vi "主动发送数据生成Condition(子VI).vi"(7 "结束时间":timestamp, 8 "数据发送协议":enum16{"2005-212协议", "2017-212协议"}(ring)=enum."2017-212协议", 9 "database":string, 10 "Label.Text":string, 11 "数值":i32) -> (0 "date/time string":string, 1 "database溢出":bool, 2 "columns":string[](array[string])=["时间", "测量模式", "数据类型", "检测值", "单位", "数据标识"], 3 "CONDITION":string)   [LabVIEW 2016, in "数据传输系统-02.lvlib"]
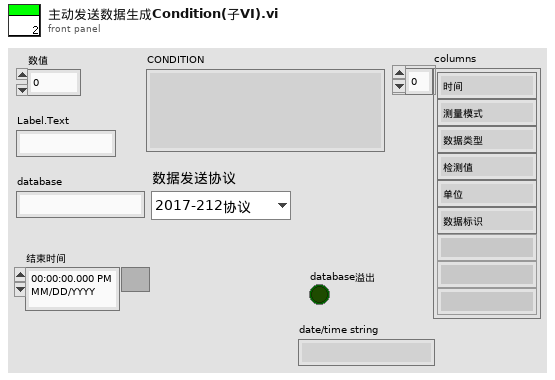
[diagram p1: front panel]
types:
  T1 = cluster{"time1":string, "time2":string, "time3":string, "time4":string, "time5":string, "time6":string, "time7":string, "time8":string, "time9":string, "time10":string, "time11":string, "time12":string, "time13":string, "time14":string, "time15":string, "time16":string, "time17":string, "time18":string, "time19":string, "time20":string, "time21":string, "time22":string, "time23":string, "time24":string, "time25":string, "time26":string, "time27":string, "time28":string, "time29":string, "time30":string, "time31":string, "time32":string, "time33":string, "time34":string, "time35":string, "time36":string, "time37":string, "time38":string, "time39":string, "time40":string, "time41":string, "time42":string, "time43":string, "time44":string, "time45":string, "time46":string, "time47":string, "time48":string, "time49":string, "time50":string, "time51":string, "time52":string, "time53":string, "time54":string, "time55":string, "time56":string, "time57":string, "time58":string, "time59":string, "time60":string, "time61":string, "time62":string, "time63":string, "time64":string, "time65":string, "time66":string, "time67":string, "time68":string, "time69":string, "time70":string, "time71":string, "time72":string, "time73":string, "time74":string, "time75":string, "time76":string}
  T2 = typedef "LVDateTimeRec.ctl" = cluster{"秒数的小数部分":dbl, "秒":i32, "分":i32, "时":i32, "日":i32, "月":i32, "年":i32, "天数（周）":i32, "天数（年）":i32, "DST":i32}
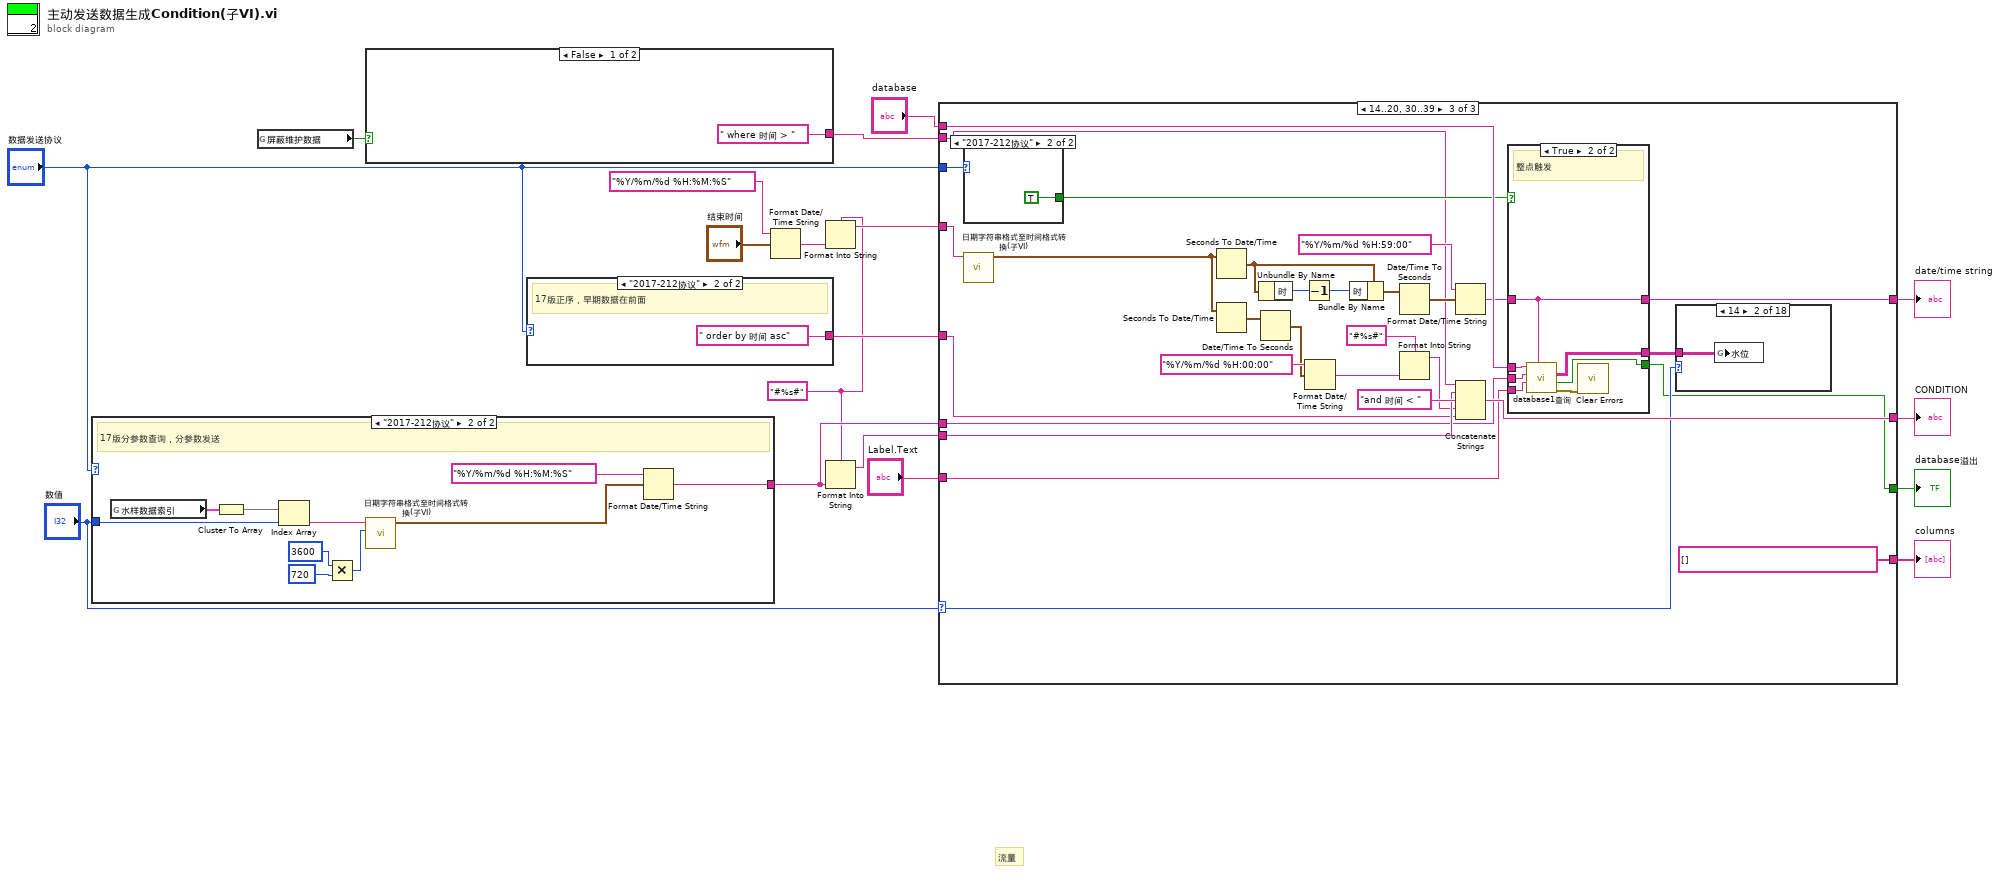
[diagram p0: block diagram]
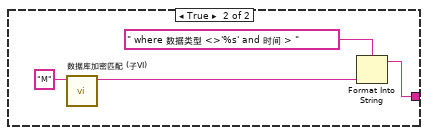
[diagram p2: hidden frame]
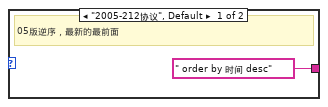
[diagram p3: hidden frame]
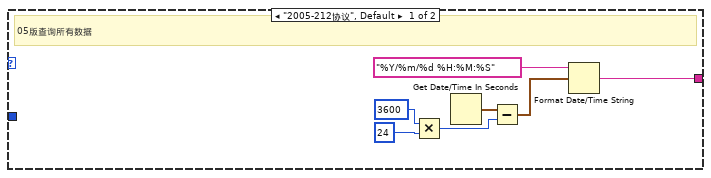
[diagram p4: hidden frame]
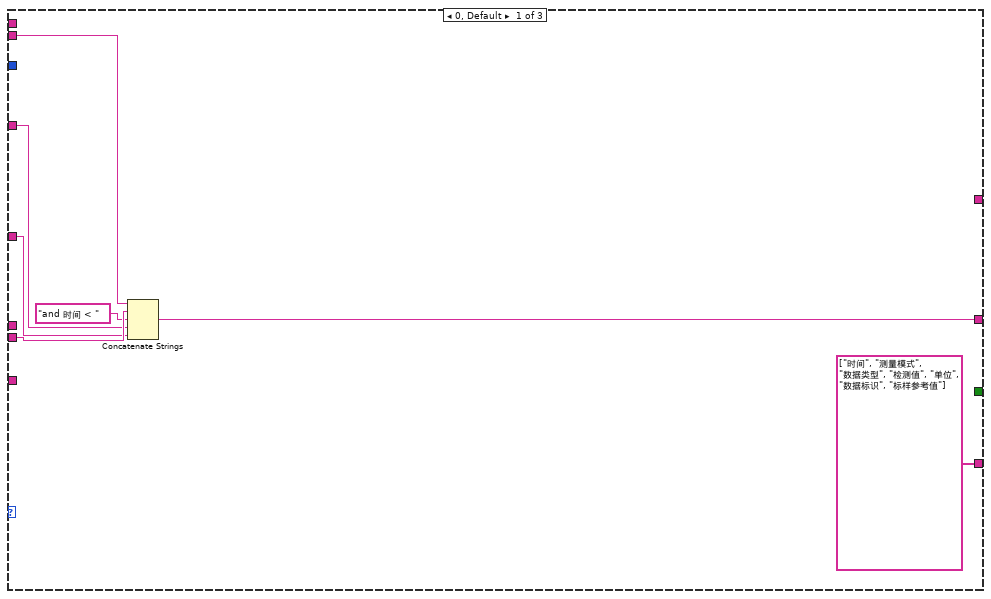
[diagram p5: hidden frame]
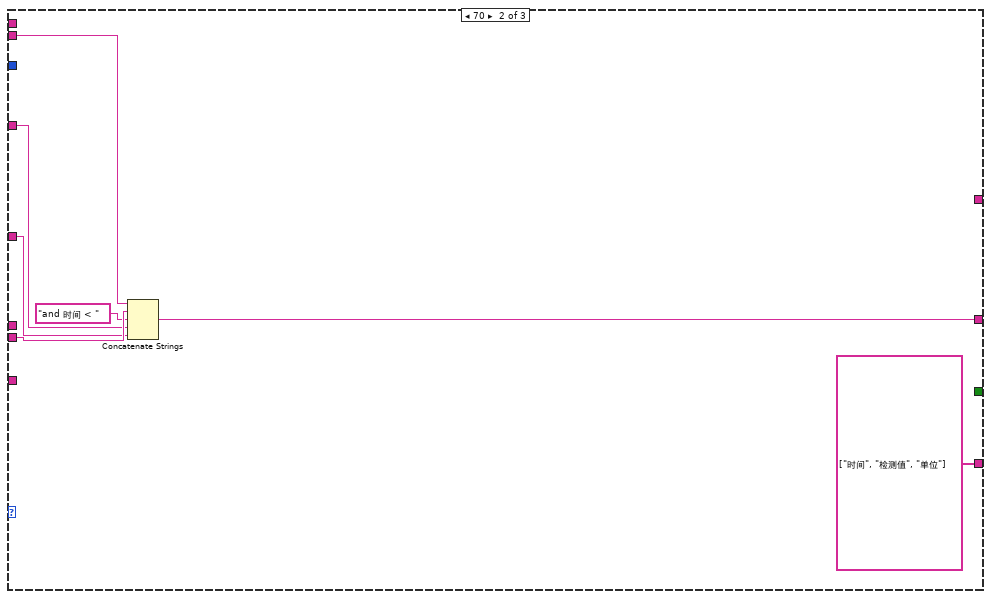
[diagram p6: hidden frame]
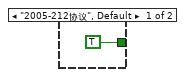
[diagram p7: hidden frame]
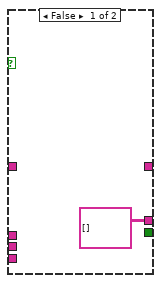
[diagram p8: hidden frame]
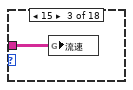
[diagram p10: hidden frame]
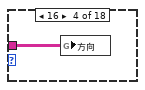
[diagram p11: hidden frame]
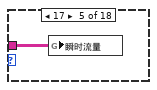
[diagram p12: hidden frame]
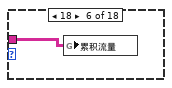
[diagram p13: hidden frame]
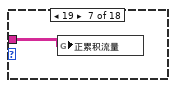
[diagram p14: hidden frame]
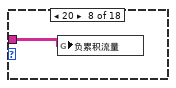
[diagram p15: hidden frame]
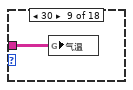
[diagram p16: hidden frame]
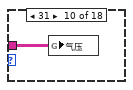
[diagram p17: hidden frame]
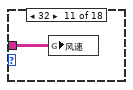
[diagram p18: hidden frame]
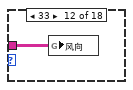
[diagram p19: hidden frame]
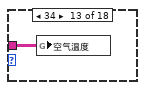
[diagram p20: hidden frame]
diagram:
  w6 = "#%s#" ("初始字符串")
  # "流量"
  n1 = case shown="\"2017-212协议\"" "数据发送协议" {
    tunnel: [w24 w27] -> w18
    tunnel: "数值" -> [_ w33]
    frame "2005-212协议", Default {
      # "05版查询所有数据"
      n2 = Multiply(x=3600, y=24) -> (x*y=w19:i32)
      n3 = Get Date/Time In Seconds() -> (seconds since 1Jan1904=w23:timestamp)
      n4 = Subtract(x=w23, y=w19) -> (x-y=w22:timestamp)
      n5 = Format Date/Time String(time format string (%c)="%Y/%m/%d %H:%M:%S" ("时间格式字符串(%c)"), seconds (now)=w22) -> (date/time string=w24:string)  [unwired: 1 in]
    }
    frame "2017-212协议" {
      # "17版分参数查询，分参数发送"
      n6 = global read "全局 水样时间.vi" "水样数据索引"() -> (w34:T1)
      n7 = Cluster To Array(cluster=w34) -> (array=w35:string[])
      n8 = Index Array(array=w35, index=w33) -> (element=w32:string)
      n9 = Multiply(x=3600, y=720) -> (x*y=w29:i32)
      n10 = call "日期字符串格式至时间格式转换(子VI).vi"("数值"=w29, "data[0]"=w32) -> ("time stamp"=w26:timestamp)  [unwired: 9 in]
      n11 = Format Date/Time String(time format string (%c)="%Y/%m/%d %H:%M:%S" ("时间格式字符串(%c)"), seconds (now)=w26) -> (date/time string=w27:string)  [unwired: 1 in]
    }
  }
  n12 = global read "断电保存全局.vi" "屏蔽维护数据"() -> (w4:bool)
  n13 = case shown="False" w4 {
    tunnel: [" where 时间 > " w39] -> w5
    frame False {
    }
    frame True {
      n14 = call "数据库加密匹配 (子VI).vi"("输入参数"="M") -> ("Encoded String"=w37:string)  [unwired: 10 in]
      n15 = Format Into String(format string=" where 数据类型 <>'%s' and 时间 > ", w37) -> (resulting string=w39:string)  [unwired: 2 in, 1 out]
    }
  }
  n16 = case shown="\"2017-212协议\"" "数据发送协议" {
    tunnel: [" order by 时间 desc" ("字符串") " order by 时间 asc" ("字符串")] -> w12
    frame "2005-212协议", Default {
      # "05版逆序，最新的最前面"
    }
    frame "2017-212协议" {
      # "17版正序，早期数据在前面"
    }
  }
  n17 = Format Date/Time String(time format string (%c)="%Y/%m/%d %H:%M:%S" ("时间格式字符串(%c)"), seconds (now)="结束时间") -> (date/time string=w3:string)  [unwired: 1 in]
  n18 = Format Into String(format string=w6, w3) -> (resulting string=w14:string)  [unwired: 2 in, 1 out]
  n19 = Format Into String(format string=w6, w18) -> (resulting string=w13:string)  [unwired: 2 in, 1 out]
  n20 = case shown="14..20, 30..39" "数值" {
    selector: "数值" -> [_ _ w80]
    tunnel: w13 -> [w49 w56 w84]
    tunnel: [w48 w55 w85] -> w8
    tunnel: w14 -> [w46 w53 w57]
    tunnel: "database" -> [_ _ w83]
    tunnel: "Label.Text" -> [_ _ w82]
    tunnel: w18 -> [_ _ w68]
    tunnel: w12 -> [w45 w52 w79]
    tunnel: [string[] ["时间", "测量模式", "数据类型", "检测值", "单位", "数据标识", "标样参考值"] ("columns") string[] ["时间", "检测值", "单位"] ("columns") string[] [] ("columns")] -> w11
    tunnel: "数据发送协议" -> [_ _ w76]
    tunnel: w5 -> [w43 w50 w67]
    tunnel: [_ _ w59] -> w1
    tunnel: [_ _ w58] -> w2
    frame 0, Default {
      n21 = Concatenate Strings(w43, w49, "and 时间 < " ("字符串"), w46, w45) -> (w48:string)
    }
    frame 70 {
      n22 = Concatenate Strings(w50, w56, "and 时间 < " ("字符串"), w53, w52) -> (w55:string)
    }
    frame 14..20, 30..39 {
      n23 = case shown="\"2017-212协议\"" w76 {
        tunnel: [TRUE TRUE] -> w78
        frame "2005-212协议", Default {
        }
        frame "2017-212协议" {
        }
      }
      n24 = call "日期字符串格式至时间格式转换(子VI).vi"("data[0]"=w57) -> ("time stamp"=w64:timestamp)  [unwired: 10 in]
      n25 = Seconds To Date/Time(time stamp (now)=w64) -> (date time rec=w73:T2)  [unwired: 1 in]
      n26 = Seconds To Date/Time(time stamp (now)=w64) -> (date time rec=w63:T2)  [unwired: 1 in]
      n27 = Unbundle By Name(w73) -> ("时"=w74:i32)
      n28 = Date/Time To Seconds(2:w63) -> (0:w65:timestamp)  [unwired: 1 in]
      n29 = Decrement(x=w74) -> (x-1=w75:i32)
      n30 = Format Date/Time String(time format string (%c)="%Y/%m/%d %H:00:00" ("时间格式字符串(%c)"), seconds (now)=w65) -> (date/time string=w61:string)  [unwired: 1 in]
      n31 = Bundle By Name(cluster=w73, "时"=w75) -> (w72:T2)
      n32 = Date/Time To Seconds(2:w72) -> (0:w71:timestamp)  [unwired: 1 in]
      n33 = Format Into String(format string="#%s#" ("初始字符串"), w61) -> (resulting string=w60:string)  [unwired: 2 in, 1 out]
      n34 = Format Date/Time String(time format string (%c)="%Y/%m/%d %H:59:00" ("时间格式字符串(%c)"), seconds (now)=w71) -> (date/time string=w69:string)  [unwired: 1 in]
      n35 = Concatenate Strings(w67, w84, "and 时间 < " ("字符串"), w60, w79) -> (w85:string)
      n36 = case shown="True" w78 {
        tunnel: w83 -> [_ w96]
        tunnel: w82 -> [_ w95]
        tunnel: [string[][] [] ("data") w94] -> w81
        tunnel: w69 -> [_ w91]
        tunnel: w68 -> [_ w92]
        tunnel: [_ w91] -> w59
        tunnel: [_ w90] -> w58
        frame False {
        }
        frame True {
          # "整点触发"
          n37 = call "database1查询.vi"("终止时间"=w91, "table"=w95, "起始时间"=w92, "database"=w96) -> ("error out"=w93:errorcluster, "database溢出"=w90:bool, "data"=w94:string[][])  [unwired: 4 in, 1 out]
          n38 = call <vilib>:"Clear Errors.vi"("error in (no error)"=w93) -> ()  [unwired: 5 in, 2 out]
        }
      }
      n39 = case shown="14" w80 {
        tunnel: w81 -> [_ w97 w98 w99 w100 w101 w102 w103 w104 w105 w106 w107 w108 w109 w110 w111 w112 w113]
        frame 0, Default {
        }
        frame 14 {
          n40 = global write "全局 所有参数.vi" "水位"(w97) -> ()
        }
        frame 15 {
          n41 = global write "全局 所有参数.vi" "流速"(w98) -> ()
        }
        frame 16 {
          n42 = global write "全局 所有参数.vi" "方向"(w99) -> ()
        }
        frame 17 {
          n43 = global write "全局 所有参数.vi" "瞬时流量"(w100) -> ()
        }
        frame 18 {
          n44 = global write "全局 所有参数.vi" "累积流量"(w101) -> ()
        }
        frame 19 {
          n45 = global write "全局 所有参数.vi" "正累积流量"(w102) -> ()
        }
        frame 20 {
          n46 = global write "全局 所有参数.vi" "负累积流量"(w103) -> ()
        }
        frame 30 {
          n47 = global write "全局 所有参数.vi" "气温"(w104) -> ()
        }
        frame 31 {
          n48 = global write "全局 所有参数.vi" "气压"(w105) -> ()
        }
        frame 32 {
          n49 = global write "全局 所有参数.vi" "风速"(w106) -> ()
        }
        frame 33 {
          n50 = global write "全局 所有参数.vi" "风向"(w107) -> ()
        }
        frame 34 {
          n51 = global write "全局 所有参数.vi" "空气温度"(w108) -> ()
        }
        frame 35 {
          n52 = global write "全局 所有参数.vi" "相对湿度"(w109) -> ()
        }
        frame 36 {
          n53 = global write "全局 所有参数.vi" "分钟雨量"(w110) -> ()
        }
        frame 37 {
          n54 = global write "全局 所有参数.vi" "小时雨量"(w111) -> ()
        }
        frame 38 {
          n55 = global write "全局 所有参数.vi" "日雨量"(w112) -> ()
        }
        frame 39 {
          n56 = global write "全局 所有参数.vi" "累积雨量"(w113) -> ()
        }
      }
    }
  }
  "CONDITION" <- w8
  "columns" <- w11
  "database溢出" <- w2
  "date/time string" <- w1
